vi "Get Data.vi"(5 "End (Full)":dbl, 6 "Timeout ms (1000)":i32=1000, 7 "Start (Full)":dbl, 8 "error in (no error)":errorcluster, 10 "Channels":string[](array[string]), 11 "Historian API in":refnum<class "Historian API.lvclass">) -> (0 "error out":errorcluster, 2 "History Data (LV Dbl)":T1, 3 "Historian API out":refnum<class "Historian API.lvclass">)   [LabVIEW 2020, in "VolatusHistorian.lvlib" / "Historian API.lvclass"]
uses:
  Historian API.lvclass
  Historian API.lvclass/Historian API.ctl
  Volatus/MessageQ/MessageQ.lvclass
  Data Request.ctl
  VolatusHistorian.lvlib
  Local Data Value/LV Dbl Data Value.lvclass
  C:/dev/lv20CE/relink/lv-promises/Promises/Value/Value.lvclass
  C:/dev/lv20CE/relink/lv-volatus/VolatusHistorian/Local Data Value/LV Dbl Data Value.lvclass
  Channel History (LV Dbl).ctl
  History Data (LV Dbl).ctl
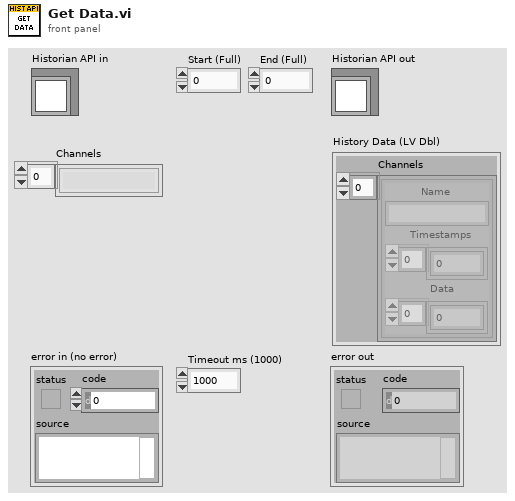
[diagram p1: front panel]
types:
  T1 = typedef "VolatusHistorian.lvlib/History Data (LV Dbl).ctl" = cluster{"Channels":T2[]}
  T2 = typedef "VolatusHistorian.lvlib/Channel History (LV Dbl).ctl" = cluster{"Name":string, "Timestamps":dbl[], "Data":dbl[]}
  T3 = typedef "VolatusHistorian.lvlib/Data Request.ctl" = cluster{"Channels":string[], "Start Time":dbl, "End Time":dbl}
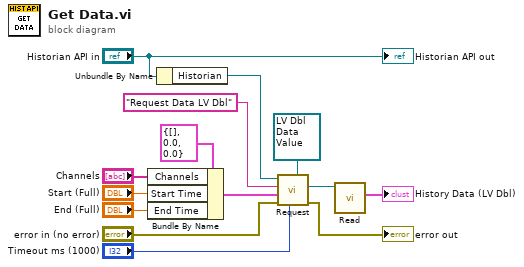
[diagram p0: block diagram]
diagram:
  n1 = Bundle By Name(cluster=T3 {"Channels"=[], "Start Time"=0.0, "End Time"=0.0} ("Data Request"), "Channels"="Channels", "Start Time"="Start (Full)", "End Time"="End (Full)") -> (w10:T3)
  n2 = Unbundle By Name("Historian API in") -> ("Historian"=w8:refnum<class "MessageQ.lvclass">)
  n3 = call "Request.vi"("Response Value Type"=refnum<class "LV Dbl Data Value.lvclass"> refnum ("VolatusHistorian.lvlib:LV Dbl Data Value.lvclass"), "Timeout ms (1000)"="Timeout ms (1000)", "error in (no error)"="error in (no error)", "Data"=w10, "ID"="Request Data LV Dbl", "MessageQ in"=w8) -> ("error out"=→"error out":errorcluster, "Response"=w3:refnum<class "LV Dbl Data Value.lvclass">)  [unwired: 3 in, 1 out]
  n4 = call "Read.vi"("Local Data Value in"=w3) -> ("Data"=→"History Data (LV Dbl)":T1)  [unwired: 10 in]
  "Historian API out" <- "Historian API in"
